vi "ClassHierarchy.vi"(8 "error in (no error)":errorcluster, 11 "Object in":refnum<class "OpenG_Value_Object.lvclass">) -> (0 "error out":errorcluster, 2 "Class hierarchy":string[](array[string]), 3 "Object out":refnum<class "OpenG_Value_Object.lvclass">)   [LabVIEW 2015, in "OpenG_Value_Object.lvclass"]
doc: "Returns the class hierarchy of an object."
uses:
  <userlib>/_OpenG.lib/openg_object/openg_value_object.llb/OpenG_Value_Object.lvclass
  <userlib>/_OpenG.lib/openg_object/openg_object.llb/OpenG_Object.lvclass
panel:
  # "Please visit http://www.OpenG.org to learn about the\nOpen Source LabVIEW software movement.\n\nNOTICE -- YOU MUST LEAVE THIS NOTICE IN PLACE.  PER THE TERMS OF THE LICENSE BELOW, YOU MAY SUBLICENSE THIS SOFTWARE \nIN ANY WAY THAT DOES NOT CONFLICT WITH THIS LICENSE.\n\n### BSD License (http://www.opensource.org/licenses/bsd-license.php) Begin ###\n\nCopyright (c) 2007, Tomi Maila\nCopyright (c) 2007, Endevo AB\n\n\nAll rights reserved.\n\nRedistribution and use in source and binary forms, with or without modification, are permitted provided that the following conditions are met:\n\n    * Redistributions of source code must retain the above copyright notice, this list of conditions and the following disclaimer.\n    * Redistributions in binary form must reproduce the above copyright notice, this list of conditions and the following disclaimer in the \n       documentation and/or other materials provided with the distribution.\n    * Neither the name of Endevo AB nor the names of the contributors may be used to endorse or promote products derived\n       from this software without specific prior written permission.\n\nTHIS SOFTWARE IS PROVIDED BY THE COPYRIGHT HOLDERS AND CONTRIBUTORS \"AS IS\" AND ANY EXPRESS OR IMPLIED WARRANTIES, \nINCLUDING, BUT NOT LIMITED TO, THE IMPLIED WARRANTIES OF MERCHANTABILITY AND FITNESS FOR A PARTICULAR PURPOSE ARE \nDISCLAIMED. IN NO EVENT SHALL THE COPYRIGHT OWNER OR CONTRIBUTORS BE LIABLE FOR ANY DIRECT, INDIRECT, INCIDENTAL,\n SPECIAL, EXEMPLARY, OR CONSEQUENTIAL DAMAGES (INCLUDING, BUT NOT LIMITED TO, PROCUREMENT OF SUBSTITUTE GOODS OR \nSERVICES; LOSS OF USE, DATA, OR PROFITS; OR BUSINESS INTERRUPTION) HOWEVER CAUSED AND ON ANY THEORY OF LIABILITY, \nWHETHER IN CONTRACT, STRICT LIABILITY, OR TORT (INCLUDING NEGLIGENCE OR OTHERWISE) ARISING IN ANY WAY OUT OF THE USE \nOF THIS SOFTWARE, EVEN IF ADVISED OF THE POSSIBILITY OF SUCH DAMAGE.\n\n### BSD License End ###"
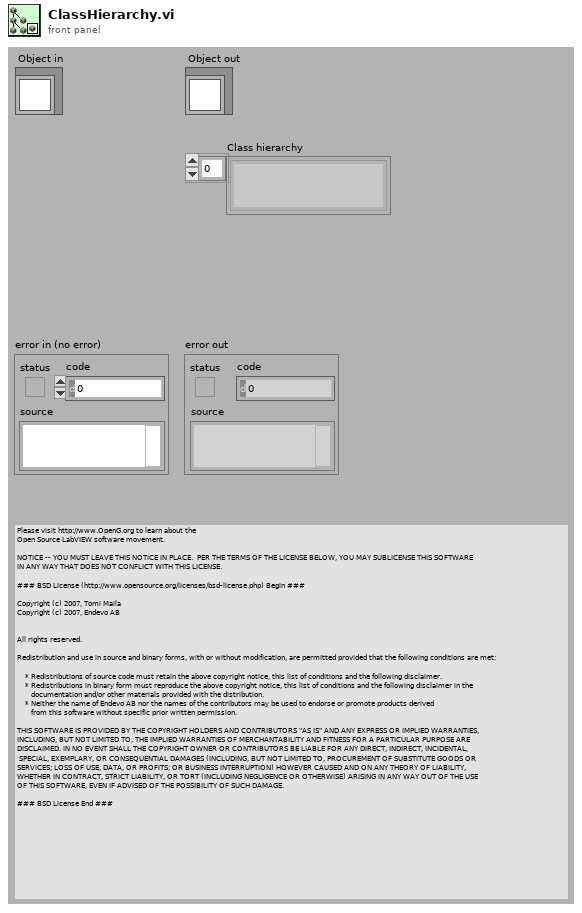
[diagram p1: front panel]
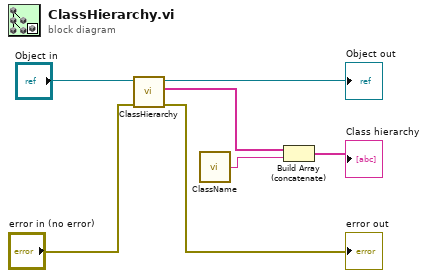
[diagram p0: block diagram]
diagram:
  n1 = call-parent "ClassHierarchy.vi"("error in (no error)"="error in (no error)", "Object in"="Object in") -> ("error out"=→"error out":errorcluster, "Class hierarchy"=w1:string[], "Object out"=→"Object out":refnum<class "OpenG_Value_Object.lvclass">)  [unwired: 7 in]
  n2 = call <userlib>:"ClassName.vi"() -> ("class name"=w6:string)  [unwired: 1 in]
  n3 = Build Array (concatenate)(w1, w6) -> (→"Class hierarchy":string[])
